vi "Initialize Sweep Channels.vi"(8 "error in (no error)":errorcluster, 11 "Instrument.DAQ":refnum<class "Instrument.DAQ.lvclass">) -> (0 "error out":errorcluster, 3 "Instrument.DAQ out":refnum<class "Instrument.DAQ.lvclass">)   [LabVIEW 2019, in "Instrument.Lockin.lvlib" / "Instrument.DAQ.lvclass"]
uses:
  Instrument.DAQ.lvclass
  Instrument.DAQ.lvclass/Instrument.DAQ.ctl
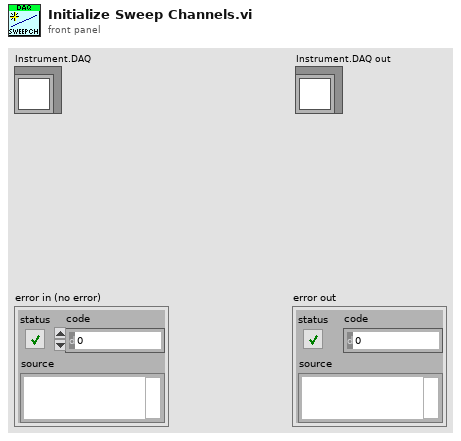
[diagram p1: front panel]
types:
  T1 = typedef "Instrument.Lockin.lvlib/Instrument.DAQ.lvclass/Sweep.Channel--Cluster--Array.ctl" = T2[]
  T2 = typedef "Instrument.Lockin.lvlib/Instrument.DAQ.lvclass/Sweep.Channel--Cluster.ctl" = cluster{"Enable?":bool, "Channel":u16, "Start":dbl, "End":dbl, "Pattern":T3, "Table":dbl[]}
  T3 = typedef "Instrument.Lockin.lvlib/Instrument.DAQ.lvclass/Sweep.Pattern--Enum.ctl" = enum16{"Ramp /", "Ramp /\\", "Smooth Ramp _/", "Smooth Ramp _/\\_", "Table"}
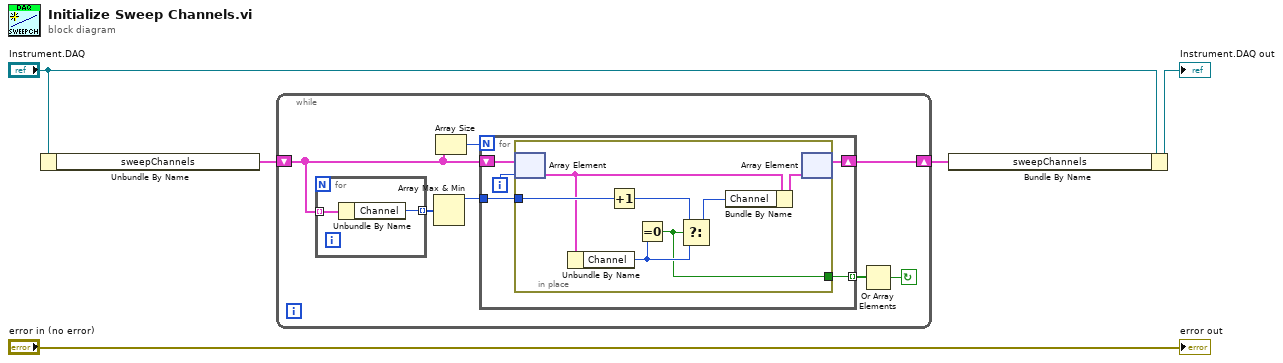
[diagram p0: block diagram]
diagram:
  n1 = Unbundle By Name("Instrument.DAQ") -> ("sweepChannels"=w2:T1)
  n2 = while {
    shift-right: [w10] -> w1
    shift-left: w2 -> [w6]
    stop <- w8 continue-if-true
    n3 = for {
      tunnel: w6 -> [w13] mode=indexing
      tunnel: [w14] -> w12 mode=indexing
      n4 = Unbundle By Name(w13) -> ("Channel"=w14:u16)
    }
    n5 = Array Max & Min(array=w12) -> (max value=w11:u16)  [unwired: 3 out]
    n6 = Array Size(array=w6) -> (size(s)=w7:i32)
    n7 = for {
      N: w7 -> [_]
      tunnel: w11 -> [w19]
      tunnel: [w18] -> w9 mode=indexing
      shift-right: [w17] -> w10
      shift-left: w6 -> [w16]
      i -> [w15]
      n8 = in-place {
        in-place-border: w19 -> [w26]
        in-place-border: [w20] -> w18
        n9 = in-place-array #1(w16, w15) -> (w21:T2)
        n10 = Unbundle By Name(w21) -> ("Channel"=w23:u16)
        n11 = Increment(x=w26) -> (x+1=w24:u16)
        n12 = Equal To 0?(x=w23) -> (x = 0?=w20:bool)
        n13 = Select(t=w24, s=w20, f=w23) -> (s? t:f=w25:u16)
        n14 = Bundle By Name(cluster=w21, "Channel"=w25) -> (w22:T2)
        n15 = in-place-array #1(w22) -> (w17:T1)  [unwired: 1 out]
      }
    }
    n16 = Or Array Elements(Boolean array=w9) -> (logical OR=w8:bool)
  }
  n17 = Bundle By Name(cluster="Instrument.DAQ", "sweepChannels"=w1) -> (→"Instrument.DAQ out":refnum<class "Instrument.DAQ.lvclass">)
  "error out" <- "error in (no error)"
